vi "Test Case Error or No Error.vi"() -> ()   [LabVIEW 2017]
uses:
  JSONtext.lvlib
  <vilib>/addons/_JKI Toolkits/Caraya/classes/Test/Test.lvclass
  <vilib>/addons/_JKI Toolkits/Caraya/classes/Assert/Assert.lvclass
panel:
  out "Equals":bool[](array[boolean])
  out "Test Cases results 2":string[](array[string])
  out "Should be Error":errorcluster[](array[cluster])
  out "Should be no Error":errorcluster[](array[cluster])
  out "Test Cases results":string[](array[string])
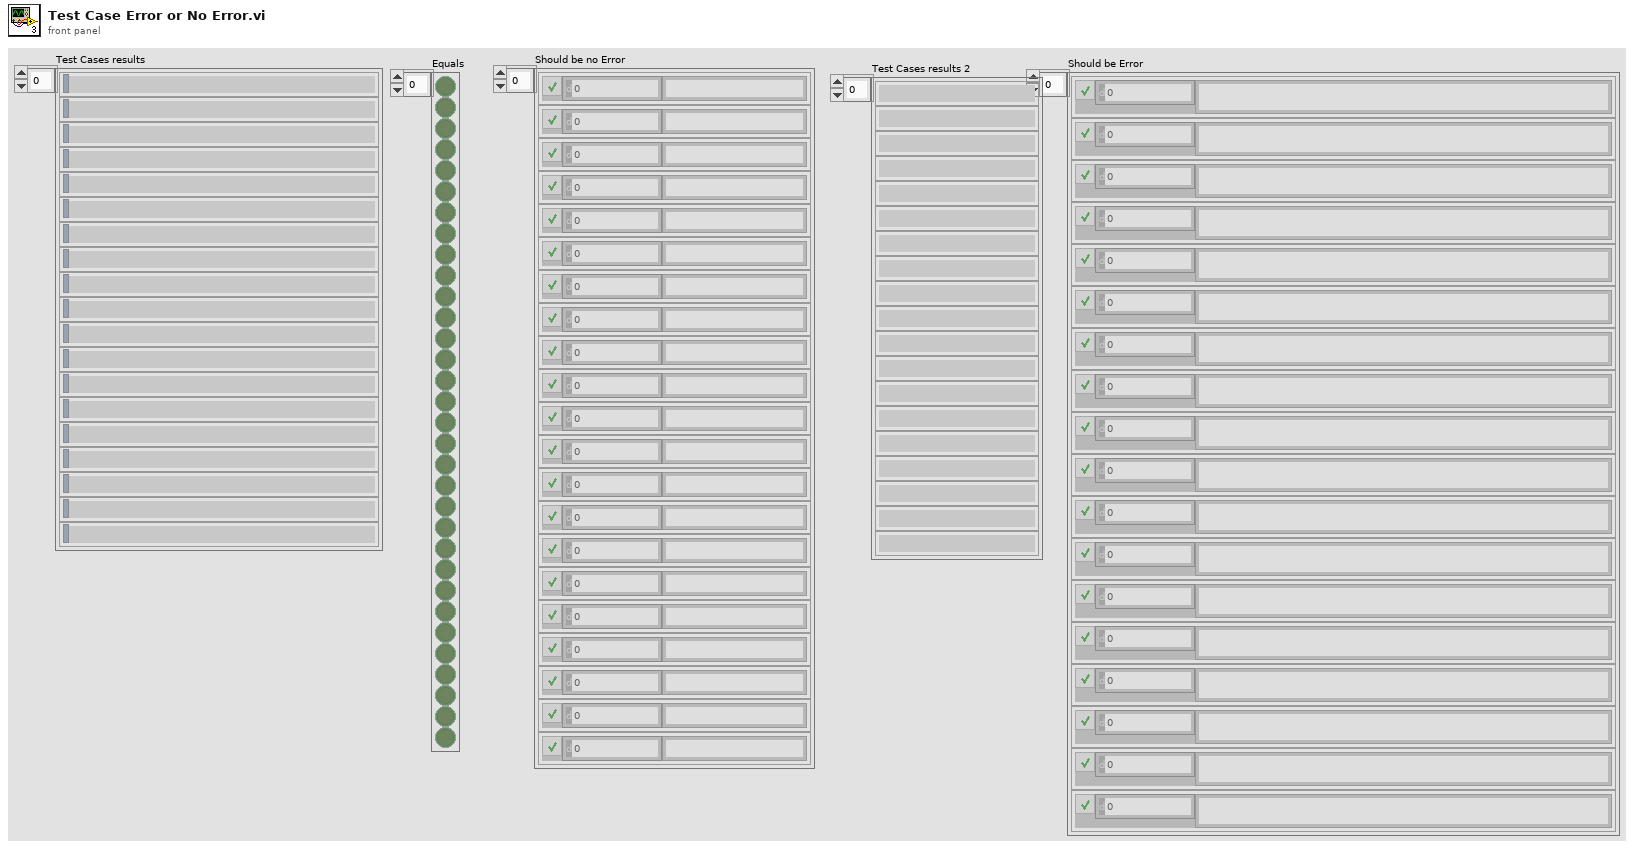
[diagram p1: front panel]
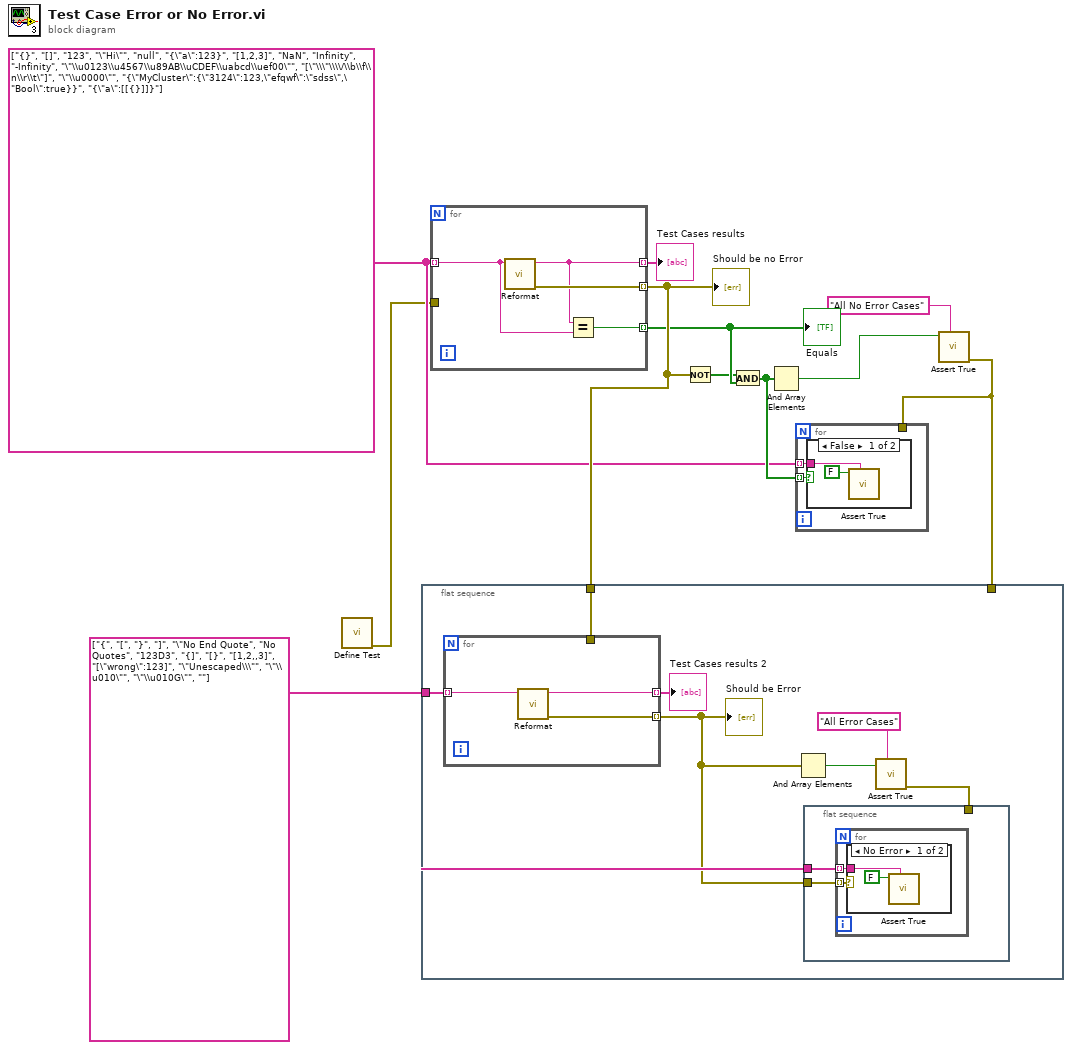
[diagram p0: block diagram]
diagram:
  w3 = string[] ["{}", "[]", "123", "\"Hi\"", "null", "{\"a\":123}", "[1,2,3]", "NaN", "Infinity", "-Infinity", "\"\\u0123\\u4567\\u89AB\\uCDEF\\uabcd\\uef00\"", "[\"\\\"\\\\/\\b\\f\\n\\r\\t\"]", "\"\\u0000\"", "{\"MyCluster\":{\"3124\":123,\"efqwf\":\"sdss\",\"Bool\":true}}", "{\"a\":[[{}]]}"]
  n1 = call <vilib>:"Define Test.vi"() -> ("error out"=w2:errorcluster)  [unwired: 11 in]
  n2 = flat-sequence {
    tunnel: w10 -> [w17]
    tunnel: string[] ["{", "[", "}", "]", "\"No End Quote", "No Quotes", "123D3", "{]", "[}", "[1,2,,3]", "[\"wrong\":123]", "\"Unescaped\\\"", "\"\\u010\"", "\"\\u010G\"", ""] -> [w14]
    tunnel: w1 -> [_]
    frame #0 {
      n3 = for {
        tunnel: w14 -> [w27] mode=indexing
        tunnel: [w26] -> w18 mode=indexing
        tunnel: [w25] -> w13 mode=indexing
        tunnel: w17 -> [_]
        n4 = call "Reformat.vi"("JSON"=w27) -> ("error out"=w25:errorcluster, "<JSON>First JSON Value\n\n<JSON>"=w26:string)  [unwired: 7 in, 2 out]
      }
      "Test Cases results 2" <- w18
      "Should be Error" <- w13
      n5 = And Array Elements(Boolean array=w13) -> (logical AND=w15:bool)
      n6 = flat-sequence {
        tunnel: w14 -> [w20]
        tunnel: w13 -> [w19]
        tunnel: w12 -> [_]
        frame #0 {
          n7 = for {
            tunnel: w20 -> [w22] mode=indexing
            tunnel: w19 -> [w21] mode=indexing
            n8 = case shown="No Error" w21 {
              tunnel: w22 -> [w24 _]
              frame No Error {
                n9 = call <vilib>:"Assert True.vi"("Label"=w24, "True?"=FALSE) -> ()  [unwired: 9 in, 1 out]
              }
              frame Error {
              }
            }
          }
        }
      }
      n10 = call <vilib>:"Assert True.vi"("Label"="All Error Cases", "True?"=w15) -> ("error out"=w12:errorcluster)  [unwired: 9 in]
    }
  }
  n11 = for {
    tunnel: w3 -> [w29] mode=indexing
    tunnel: [w30] -> w11 mode=indexing
    tunnel: [w31] -> w10 mode=indexing
    tunnel: [w28] -> w9 mode=indexing
    tunnel: w2 -> [_]
    n12 = call "Reformat.vi"("JSON"=w29) -> ("error out"=w31:errorcluster, "<JSON>First JSON Value\n\n<JSON>"=w30:string)  [unwired: 7 in, 2 out]
    n13 = Equal?(x=w30, y=w29) -> (x = y?=w28:bool)
  }
  "Test Cases results" <- w11
  "Should be no Error" <- w10
  "Equals" <- w9
  n14 = Not(x=w10) -> (.not. x?=w8:bool[])
  n15 = And(x=w8, y=w9) -> (x .and. y?=w4:bool[])
  n16 = And Array Elements(Boolean array=w4) -> (logical AND=w6:bool)
  n17 = call <vilib>:"Assert True.vi"("Label"="All No Error Cases", "True?"=w6) -> ("error out"=w1:errorcluster)  [unwired: 9 in]
  n18 = for {
    tunnel: w3 -> [w33] mode=indexing
    tunnel: w4 -> [w32] mode=indexing
    tunnel: w1 -> [_]
    n19 = case shown="False" w32 {
      tunnel: w33 -> [w35 _]
      frame False {
        n20 = call <vilib>:"Assert True.vi"("Label"=w35, "True?"=FALSE) -> ()  [unwired: 9 in, 1 out]
      }
      frame True {
      }
    }
  }
